vi "Send Shortcut Menu Activation.vi"(0 "Message Enqueuer in":refnum<class "Message Enqueuer.lvclass">, 3 "EventFilter Reference":T1, 5 "CtlRef":refnum<vi>, 7 "Time":u32, 9 "MenuRef":refnum<k9>, 11 "Coords":T2, 12 "SubObj":refnum<vi>) -> (4 "Filtered EventDataMessage":refnum<class "ShortcutMenuActivationMsg.lvclass">, 15 "error out":errorcluster)   [LabVIEW 2018, in "MVA Framework.lvlib" / "ActorEvents.lvlib" / "ShortcutMenuActivationMsg.lvclass"]
doc: "<License>\nCopyright © 2017 Composed Systems, LLC | All rights reserved\nwww.composed.io\n\nAuthor: Ethan Stern <ethan.stern@composed.io>\n\nThis software is provided \"AS IS\" WITHOUT WARRANTIES, either express or implied, AND IS FOR EDUCATIONAL PURPOSES ONLY.\n</License>"
uses:
  ShortcutMenuActivationMsg.lvclass
  EventDataMessage/EventDataMessage.lvclass
  <vilib>/ActorFramework/Message Enqueuer/Message Enqueuer.lvclass
  <vilib>/Utility/miscctls.llb/LVPoint32TypeDef.ctl
  IEventFilter/IEventFilter.lvclass
  IEventFilter/EventFilter Reference.ctl
panel:
  in  "error in (no error)":errorcluster
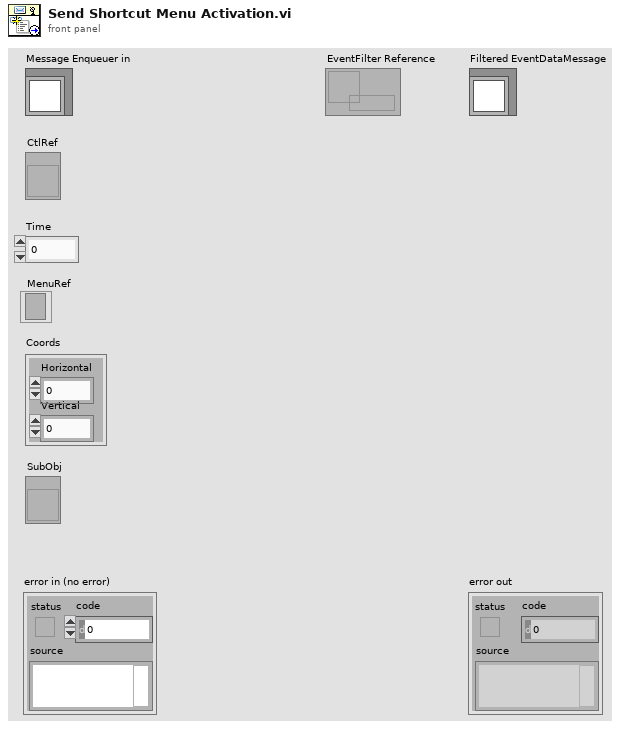
[diagram p1: front panel]
types:
  T1 = typedef "MVA Framework.lvlib/ActorEvents.lvlib/IEventFilter.lvclass/EventFilter Reference.ctl" = refnum<data-value>
  T2 = typedef "LVPoint32TypeDef.ctl" = cluster{"Horizontal":i32, "Vertical":i32}
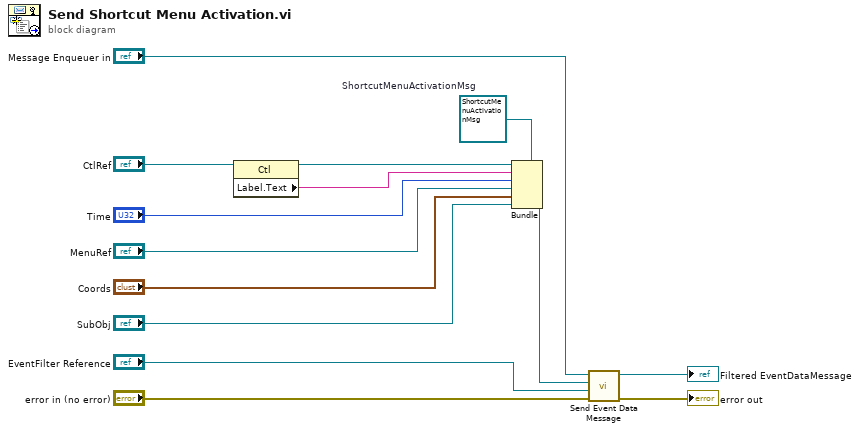
[diagram p0: block diagram]
diagram:
  w14 = refnum<class "ShortcutMenuActivationMsg.lvclass"> refnum  # ShortcutMenuActivationMsg
  n1 = property class="Ctl"(reference="CtlRef") -> (reference out=w8:refnum<vi>, "Label.Text"=w6:string)  [unwired: 1 in, 1 out]
  n2 = Bundle(cluster=w14, w8, w6, "Time", "MenuRef", "Coords", "SubObj") -> (w11:refnum<class "ShortcutMenuActivationMsg.lvclass">)
  n3 = call "Send Event Data Message.vi"("error in (no error)"="error in (no error)", "EventFilter Reference"="EventFilter Reference", "EventDataMessage"=w11, "Message Enqueuer in"="Message Enqueuer in") -> ("error out"=→"error out":errorcluster, "Filtered EventDataMessage"=→"Filtered EventDataMessage":refnum<class "ShortcutMenuActivationMsg.lvclass">)  [unwired: 6 in]
